vi "CurrentVIsParentReference.vi"() -> (3 "ParentVIReference":refnum<vi>)   [LabVIEW 2019, in "UserInterface.lvlib"]
uses:
  UserInterface.lvlib
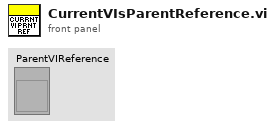
[diagram p1: front panel]
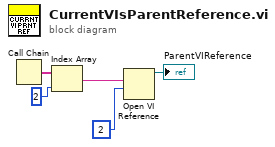
[diagram p0: block diagram]
diagram:
  n1 = Call Chain() -> (call chain=w5:string[])
  n2 = Index Array(array=w5, index=2 ("Index")) -> (element=w3:string)
  n3 = Open VI Reference(vi path=w3, options=2) -> (vi reference=→"ParentVIReference":refnum<vi>)  [unwired: 4 in, 1 out]
